vi "Set Source.vi"(0 "instrument handle in":refnum<k15>, 5 "Set Vin":string, 7 "Vin in V":dbl, 11 "error in (no error)":errorcluster) -> (4 "instrument handle out":refnum<k15>, 15 "error out":errorcluster)   [LabVIEW 2020]
uses:
  <instrlib>/niDCPower/nidcpower.llb/niDCPower Wait For Event - Event.ctl
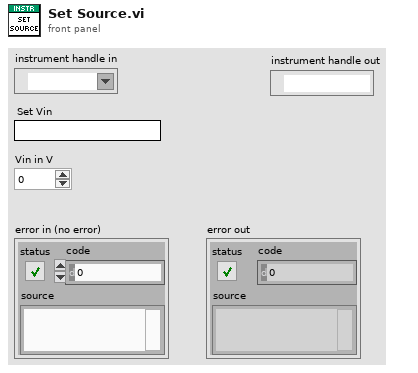
[diagram p1: front panel]
types:
  T1 = typedef "niDCPower Wait For Event - Event.ctl" = i32
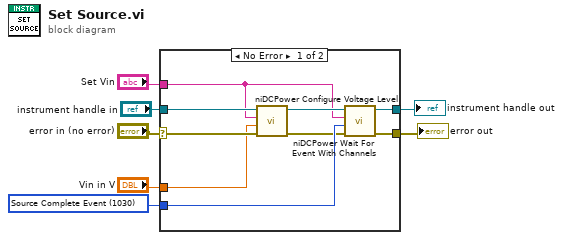
[diagram p0: block diagram]
diagram:
  w7 = T1 1030 items=["Source Complete Event"=1030, "Measure Complete Event"=1031, "Sequence Iteration Complete Event"=1032, "Sequence Engine Done Event"=1033, "Pulse Complete Event"=1051, "Ready For Pulse Trigger Event"=1052] ("event")
  n1 = case shown="No Error" "error in (no error)" {
    selector: "error in (no error)" -> [w12 w18]
    tunnel: w7 -> [w16 _]
    tunnel: [w14 w18] -> w6
    tunnel: "Set Vin" -> [w9 _]
    tunnel: "Vin in V" -> [w11 _]
    tunnel: "instrument handle in" -> [w10 w17]
    tunnel: [w8 w17] -> w1
    frame No Error {
      n2 = call <instrlib>:"niDCPower Configure Voltage Level.vi"("error in (no error)"=w12, "voltage level"=w11, "channel name"=w9, "instrument handle"=w10) -> ("error out"=w13:errorcluster, "instrument handle out"=w15:refnum<k15>)  [unwired: 6 in]
      n3 = call <instrlib>:"niDCPower Wait For Event With Channels.vi"("error in (no error)"=w13, "event"=w16, "channel name"=w9, "instrument handle"=w15) -> ("error out"=w14:errorcluster, "instrument handle out"=w8:refnum<k15>)  [unwired: 6 in]
    }
    frame Error {
    }
  }
  "error out" <- w6
  "instrument handle out" <- w1
